vi "Validate Meas Plugin Name.vi"(0 "path":path, 5 "library name":string, 11 "error in":errorcluster) -> (4 "valid name?":bool, 15 "error out":errorcluster)   [LabVIEW 2021, in "Converter.lvlib"]
uses:
  Converter.lvlib
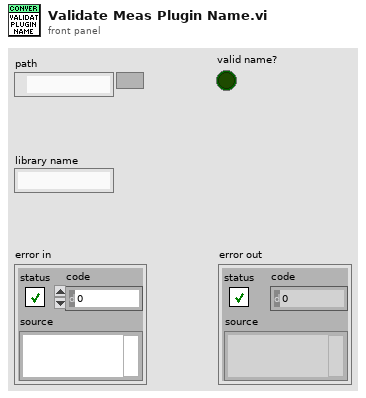
[diagram p1: front panel]
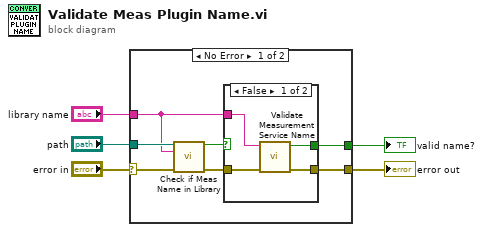
[diagram p0: block diagram]
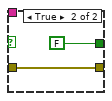
[diagram p2: hidden frame]
diagram:
  n1 = case shown="No Error" "error in" {
    selector: "error in" -> [w9 w19]
    tunnel: "path" -> [w12 _]
    tunnel: "library name" -> [w7 _]
    tunnel: [w10 _] -> w4
    tunnel: [w8 w19] -> w3
    frame No Error {
      n2 = call "Check if Meas Name in Library.vi"("path"=w12, "library name"=w7, "error in"=w9) -> ("found"=w6:bool, "error out"=w11:errorcluster)  [unwired: 11 in]
      n3 = case shown="False" w6 {
        tunnel: w11 -> [w15 w18]
        tunnel: w7 -> [w14 _]
        tunnel: [w13 FALSE ("valid name?")] -> w10
        tunnel: [w16 w18] -> w8
        frame False {
          n4 = call "Validate Measurement Service Name.vi"("error in"=w15, "requested plugin name"=w14) -> ("error out"=w16:errorcluster, "valid name?"=w13:bool)  [unwired: 8 in]
        }
        frame True {
        }
      }
    }
    frame Error {
    }
  }
  "error out" <- w3
  "valid name?" <- w4
